vi "Write PWM.vi"(0 "Left":dbl(slide) scale=0.0..1.0, 1 "Right":dbl(slide) scale=0.0..1.0) -> ()   [LabVIEW 2017]
uses:
  <vilib>/myRIO/Instrument Drivers/Onboard IO/DIO/typedefs/DIO Reference.ctl
  <vilib>/myRIO/Common/Instrument Driver Framework/Utilities/typedefs/myRIO Generic Hardware Reference.ctl
  <vilib>/myRIO/Common/Instrument Driver Framework/Utilities/typedefs/Hardware Version Enum.ctl
  <vilib>/myRIO/Common/Instrument Driver Framework/Utilities/typedefs/myRIO v1.0 Reference.ctl
  <vilib>/myRIO/Common/Instrument Driver Framework/Utilities/typedefs/Generic FPGA Reference.ctl
  <vilib>/myRIO/Common/Instrument Driver Framework/myRIO v1.0/DIO/typedefs/DIO Channels List.ctl
  <vilib>/myRIO/Common/Instrument Driver Framework/myRIO v1.0/DIO/typedefs/DIO Channels Enum.ctl
  <vilib>/userdefined/High Color/nirio_resource_hc.ctl
  <vilib>/myRIO/Instrument Drivers/Onboard IO/PWM/typedefs/PWM Reference.ctl
  <vilib>/myRIO/Common/Instrument Driver Framework/myRIO v1.0/PWM/typedefs/PWM Channels Enum.ctl
  <vilib>/myRIO/Instrument Drivers/Onboard IO/PWM/typedefs/PWM Configuration.ctl
  <vilib>/myRIO/Common/Instrument Driver Framework/Utilities/vis/Is FPGA Ref Available.vi
  <vilib>/myRIO/Common/Instrument Driver Framework/myRIO v1.0/DIO/vis/myRIO v1.1 Open DIO.vi
  <vilib>/myRIO/Instrument Drivers/Onboard IO/DIO/vis/Write.vi
  <vilib>/myRIO/Common/Instrument Driver Framework/myRIO v1.0/PWM/vis/myRIO v1.1 Open PWM.vi
  <vilib>/myRIO/Instrument Drivers/Onboard IO/PWM/vis/Set Duty Cycle and Frequency.vi
  <vilib>/myRIO/Common/Instrument Driver Framework/Utilities/vis/Validate Channels.vi
  <vilib>/myRIO/Common/Instrument Driver Framework/myRIO v1.0/DIO/vis/myRIO v1.0 Reserve DIO.vi
  <vilib>/myRIO/Common/Instrument Driver Framework/myRIO v1.0/PWM/vis/myRIO v1.0 Reserve PWM.vi
  <vilib>/myRIO/Common/Instrument Driver Framework/myRIO v1.0/Resource Manager/vis/myRIO v1.0 Reserve Channel List.vi
  <vilib>/myRIO/Common/Instrument Driver Framework/myRIO v1.0/DIO/vis/myRIO v1.0 Build MUX Configuration DIO.vi
  <vilib>/myRIO/Common/Instrument Driver Framework/myRIO v1.0/PWM/vis/myRIO v1.0 Build MUX Configuration PWM.vi
  <vilib>/myRIO/Common/Instrument Driver Framework/myRIO v1.0/Resource Manager/vis/myRIO v1.0 Reserve Channel.vi
  <vilib>/myRIO/Common/Instrument Driver Framework/myRIO v1.0/Resource Manager/vis/myRIO v1.0 Unreserve Channel.vi
  <vilib>/myRIO/Common/Instrument Driver Framework/myRIO v1.0/Resource Manager/vis/myRIO v1.0 Create Configuration List.vi
  <vilib>/myRIO/Common/Instrument Driver Framework/myRIO v1.0/Resource Manager/vis/myRIO v1.0 Build Mutex Name.vi
  <vilib>/Utility/VariantDataType/GetNumericInfo.vi
  <vilib>/Utility/error.llb/Error Cluster From Error Code.vi
  <vilib>/myRIO/Common/Instrument Driver Framework/myRIO v1.0/myRIO v1.1 Open.vi
  <vilib>/myRIO/Common/Instrument Driver Framework/Utilities/vis/IO Manager.vi
  <vilib>/myRIO/Common/Instrument Driver Framework/Utilities/vis/Configuration Manager.vi
  <vilib>/myRIO/Common/Instrument Driver Framework/myRIO v1.0/Resource Manager/vis/myRIO v1.0 Configure IO.vi
  <vilib>/myRIO/Common/Instrument Driver Framework/myRIO v1.0/myRIO v1.0 Close.vi
  <vilib>/myRIO/Common/Instrument Driver Framework/myRIO v1.0/DIO/vis/myRIO v1.0 Write DIO.vi
  <vilib>/myRIO/Express VI/Onboard IO/DO/DO Express VI.xnode
  <vilib>/myRIO/Instrument Drivers/Onboard IO/DIO/vis/myRIO DIO Open.xnode
  <vilib>/myRIO/Express VI/Onboard IO/PWM/PWM Express VI.xnode
  <vilib>/myRIO/Instrument Drivers/Onboard IO/PWM/vis/myRIO PWM Open.xnode
  <vilib>/myRIO/Instrument Drivers/Onboard IO/DIO/DIO.lvlib
  <vilib>/myRIO/Instrument Drivers/Onboard IO/PWM/PWM.lvlib
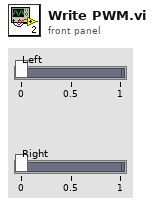
[diagram p1: front panel]
types:
  T1 = typedef "PWM.lvlib/PWM Reference.ctl" = cluster{"myRIO Reference":T2, "PWM Channels Enum":T6, "PWM Configuration":T7}
  T2 = typedef "myRIO Generic Hardware Reference.ctl" = cluster{"myRIO Model":T3, "myRIO Hardware Reference":T4}
  T3 = typedef "Hardware Version Enum.ctl" = enum16{"Unknown", "myRIO-1900", "myRIO-1950", "roboRIO", "NI ELVIS RIO CM"}
  T4 = typedef "myRIO v1.0 Reference.ctl" = cluster{"Generic FPGA Reference":T5, "Allow multiple opens":bool}
  T5 = typedef "Generic FPGA Reference.ctl" = refnum<k20>
  T6 = typedef "PWM Channels Enum.ctl" = enum16{"Not Connected", "C/PWM0", "C/PWM1", "A/PWM0", "A/PWM1", "A/PWM2", "B/PWM0", "B/PWM1", "B/PWM2", "PWM/PWM0", "PWM/PWM1", "PWM/PWM2", "PWM/PWM3", "PWM/PWM4", "PWM/PWM5", "PWM/PWM6", "PWM/PWM7", "PWM/PWM8", "PWM/PWM9"}
  T7 = typedef "PWM.lvlib/PWM Configuration.ctl" = cluster{"Frequency":dbl, "Duty Cycle":dbl}
  T8 = typedef "nirio_resource_hc.ctl" = tag
  T9 = typedef "DIO.lvlib/DIO Reference.ctl" = cluster{"myRIO Reference":T2, "DIO Channels List":T10}
  T10 = typedef "DIO Channels List.ctl" = T11[]
  T11 = typedef "DIO Channels Enum.ctl" = enum16{"Not Connected", "C/DIO0", "C/DIO1", "C/DIO2", "C/DIO3", "C/DIO4", "C/DIO5", "C/DIO6", "C/DIO7", "A/DIO0", "A/DIO1", "A/DIO2", "A/DIO3", "A/DIO4", "A/DIO5", "A/DIO6", "A/DIO7", "A/DIO8", "A/DIO9", "A/DIO10", "A/DIO11", "A/DIO12", "A/DIO13", "A/DIO14", "A/DIO15", "B/DIO0", "B/DIO1", "B/DIO2", "B/DIO3", "B/DIO4", "B/DIO5", "B/DIO6", "B/DIO7", "B/DIO8", "B/DIO9", "B/DIO10", "B/DIO11", "B/DIO12", "B/DIO13", "B/DIO14", "B/DIO15", "LED0", "LED1", "LED2", "LED3", "Button0", "DIO/DIO0", "DIO/DIO1", "DIO/DIO2", "DIO/DIO3", "DIO/DIO4", "DIO/DIO5", "DIO/DIO6", "DIO/DIO7", "DIO/DIO8", "DIO/DIO9", "SPI/CS0", "SPI/CS1", "SPI/CS2", "SPI/CS3", "LED RADIO (Green)", "LED RADIO (Red)", "LED COMM (Green)", "LED COMM (Red)", "LED MODE (Green)", "LED MODE (Red)"}
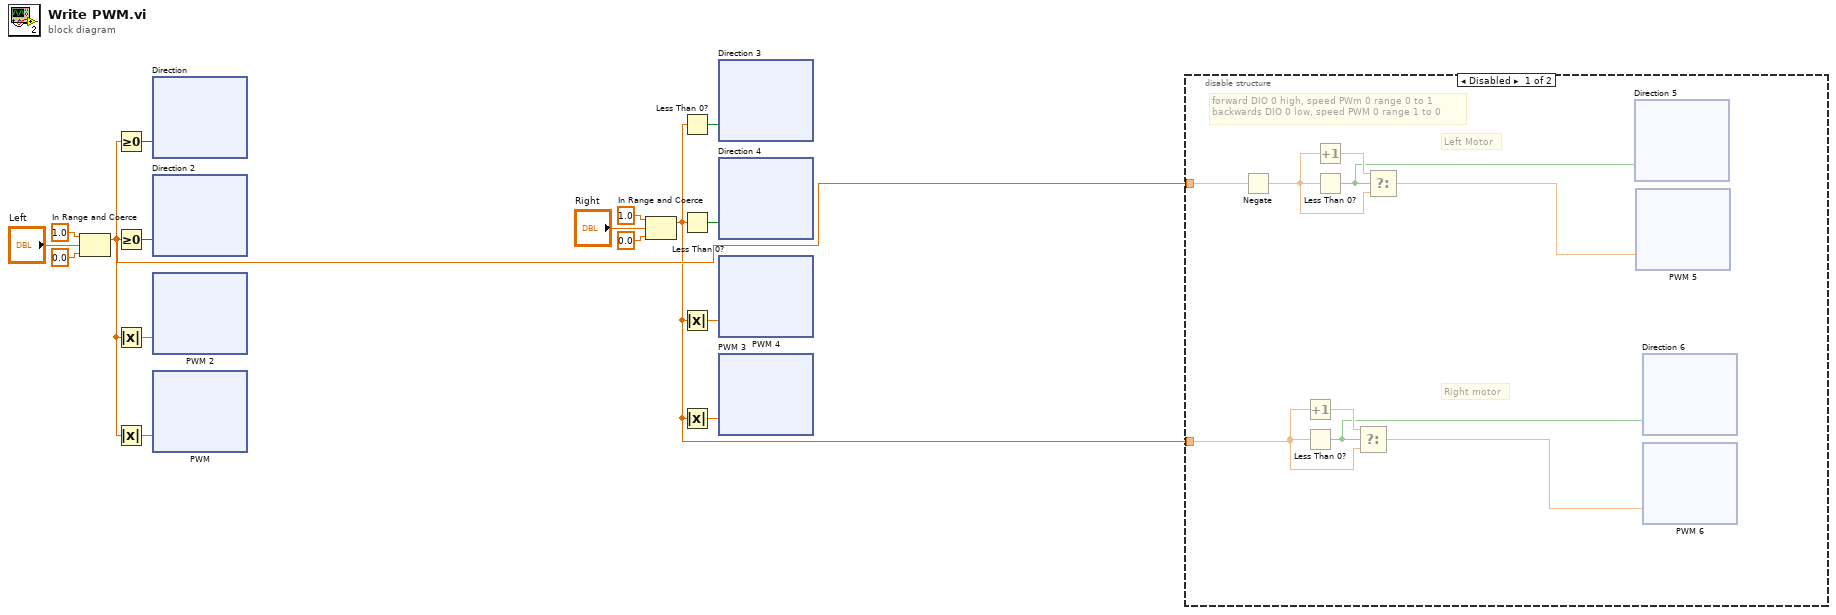
[diagram p0: block diagram]
diagram:
  n1 = In Range and Coerce(upper limit=1.0, x="Left", lower limit=0.0) -> (coerced(x)=w9:dbl)  [unwired: 1 out]
  n2 = Greater Or Equal To 0?(x=w9) -> (x >= 0?=w12:bool)
  n3 = Greater Or Equal To 0?(x=w9) -> (x >= 0?=w11:bool)
  n4 = Absolute Value(x=w9) -> (abs(x)=w16:dbl)
  n5 = Absolute Value(x=w9) -> (abs(x)=w13:dbl)
  n6 = xnode "Direction"("A/DIO3 (Pin 17)"=w12) -> ()  [unwired: 1 in, 1 out]
  n7 = xnode "Direction 2"("B/DIO4 (Pin 19)"=w11) -> ()  [unwired: 1 in, 1 out]
  n8 = xnode "PWM 2"("Duty Cycle"=w16) -> ()  [unwired: 1 in, 1 out]
  n9 = xnode "PWM"("Duty Cycle"=w13) -> ()  [unwired: 1 in, 1 out]
  n10 = In Range and Coerce(upper limit=1.0, x="Right", lower limit=0.0) -> (coerced(x)=w2:dbl)  [unwired: 1 out]
  n11 = Less Than 0?(x=w2) -> (x < 0?=w1:bool)
  n12 = Less Than 0?(x=w2) -> (x < 0?=w3:bool)
  n13 = Absolute Value(x=w2) -> (abs(x)=w15:dbl)
  n14 = Absolute Value(x=w2) -> (abs(x)=w14:dbl)
  n15 = xnode "Direction 3"("A/DIO4 (Pin 19)"=w1) -> ()  [unwired: 1 in, 1 out]
  n16 = xnode "Direction 4"("B/DIO3 (Pin 17)"=w3) -> ()  [unwired: 1 in, 1 out]
  n17 = xnode "PWM 4"("Duty Cycle"=w15) -> ()  [unwired: 1 in, 1 out]
  n18 = xnode "PWM 3"("Duty Cycle"=w14) -> ()  [unwired: 1 in, 1 out]
  n19 = disable-structure shown="Disabled" {
    disable-tunnel: w9 -> [w18 _]
    disable-tunnel: w2 -> [w17 _]
    frame Disabled {
      # "Left Motor"
      # "Right motor"
      # "forward DIO 0 high, speed PWm 0 range 0 to 1\nbackwards DIO 0 low, speed PWM 0 range 1 to 0"
      n20 = Negate(x=w18) -> (-x=w23:dbl)
      n21 = Increment(x=w17) -> (x+1=w21:dbl)
      n22 = Less Than 0?(x=w17) -> (x < 0?=w19:bool)
      n23 = Increment(x=w23) -> (x+1=w24:dbl)
      n24 = Less Than 0?(x=w23) -> (x < 0?=w22:bool)
      n25 = Select(t=w21, s=w19, f=w17) -> (s? t:f=w20:dbl)
      n26 = Select(t=w24, s=w22, f=w23) -> (s? t:f=w25:dbl)
      n27 = xnode "Direction 5"("A/DIO8 (Pin 27)"=w22) -> ()  [unwired: 1 in, 1 out]
      n28 = xnode "PWM 5"("Duty Cycle"=w25) -> ()  [unwired: 1 in, 1 out]
      n29 = xnode "Direction 6"("B/DIO8 (Pin 27)"=w19) -> ()  [unwired: 1 in, 1 out]
      n30 = xnode "PWM 6"("Duty Cycle"=w20) -> ()  [unwired: 1 in, 1 out]
    }
    frame Enabled {
    }
  }
